vi "Assemble-image-sizes-array.vi"(8 "error in":errorcluster, 9 "ROI height [pixels]":u32, 10 "ROI width [pixels]":u32, 11 "Number of cameras":i32) -> (0 "error IO":errorcluster, 2 "Image sizes":u32[][](array[numeric]))   [LabVIEW 2013, in "CameraVision.lvlib" / "CV-Configuration.lvclass"]
uses:
  CV-Configuration.lvclass
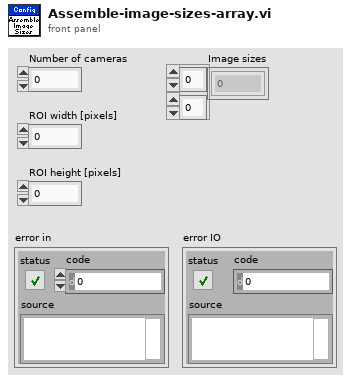
[diagram p1: front panel]
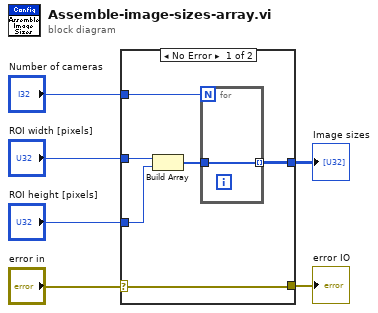
[diagram p0: block diagram]
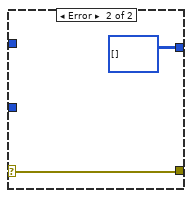
[diagram p2: hidden frame]
diagram:
  n1 = case shown="No Error" "error in" {
    selector: "error in" -> [w7 w15]
    tunnel: [w12 u32[][] []] -> w6
    tunnel: "Number of cameras" -> [w10 _]
    tunnel: "ROI height [pixels]" -> [w9 _]
    tunnel: "ROI width [pixels]" -> [w8 _]
    tunnel: [w7 w15] -> w1
    frame No Error {
      n2 = Build Array(w8, w9) -> (w11:u32[])
      n3 = for {
        N: w10 -> [_]
        tunnel: w11 -> [w13]
        tunnel: [w13] -> w12 mode=indexing
      }
    }
    frame Error {
    }
  }
  "Image sizes" <- w6
  "error IO" <- w1
